vi "RotationApplication v5.vi"() -> ()   [LabVIEW 2012]
uses:
  <instrlib>/ZaberTSeries/Public/Utility/Request.ctl
  <instrlib>/ZaberTSeries/Public/Utility/Response.ctl
  <vilib>/Utility/file.llb/Write To Spreadsheet File (string).vi
  variables/GlobalUI.vi
  Stage Global.vi
  <instrlib>/ZaberTSeries/ZaberTSeries.lvlib
panel:
  out "Scanning?":bool
  out "Current Angle (deg)":dbl=45.0
  out "Stage Position (mm)":dbl=76.5
  in  "Time Step (ms)":dbl
  in  "Rotation f(x) (mm -> deg)":string="9.00000*x - 643.50000"
  in  "Finish Rotation f(x)":bool
  in  "Scan":bool
  in  "stop":bool
  in  "Go Home":bool
  in  "Set Home Offset":dbl=80.0
  in  "?":T1(tab)
  in  "Optimize":bool
  in  "Angle?":bool
  out "Current Angle (deg)":dbl=52.314375
  in  "Move Rel?":bool
  in  "Move Abs?":bool
  in  "Move Rel (deg)":dbl=-1.0 step=0.1
  in  "Move Abs (deg)":dbl=35.0
  in  "Send":bool
  out "Command?":bool=TRUE
  in  "REQUEST:":T2={"Device Number"=1, "Command"=23, "Data"=-10000, "Response Count"=1} {"Command" items=["Echo"=55, "Home"=1, "Move Absolute"=20, "Move Relative"=21, "Move at Constant Speed"=22, "Renumber"=2, "Restore Settings"=36, "Stop"=23]}
  out "Response Data:":T3 {"Command" items=["Constant Speed Tracking"=8, "Echo"=55, "Error"=255, "Home"=1, "Limit Active"=9, "Manual Move Tracking"=10, "Move Absolute"=20, "Move at Constant Speed"=22, "Move Relative"=21, "Renumber"=2, "Restore Settings"=36, "Stop"=23]}
  in  "Command":bool
  in  "DONE":bool
  in  "angle":dbl=7.89375
  in  "Aquire Data":bool
  out "Intensity vs Angle Plot":cluster{dbl[], dbl[]}(graph)={[0.1003125, 0.200625, 0.30093749999999997, 0.40125, 0.5015625, 0.6018749999999999, 0.7021875, 0.8025, 0.9028125, 1.003125, 1.1034374999999998, 1.2037499999999999, 1.3040625, 1.404375, 1.5046875, 1.605, 1.7053125, 1.805625, 1.9059374999999998, 2.00625, 2.1065625, 2.2068749999999997, 2.3071875, 2.4074999999999998, 2.5078125, 2.608125, 2.7084375, 2.80875, 2.9090625, 3.009375, 3.1096874999999997, 3.21, 3.3103124999999998, 3.410625, 3.5109375, 3.61125, 3.7115625, 3.8118749999999997, 3.9121875, 4.0125, 4.1128124999999995, 4.213125, 4.3134375, 4.413749999999999], [0.10330483041158461, 0.10354301638719464, 0.10354301638719464, 0.10358827172256029, 0.10358827172256029, 0.10288562309451152, 0.10288562309451152, 0.10288562309451152, 0.1017709127286577, 0.1017709127286577, 0.10044183498475528, 0.09877691501524301, 0.09877691501524301, 0.10001548208841382, 0.10001548208841382, 0.09941763528963352, 0.09941763528963352, 0.09897222751524294, 0.09965820312499914, 0.09965820312499914, 0.09993807164634047, 0.09985708841463325, 0.09985708841463325, 0.09985708841463325, 0.10042158917682856, 0.10075624047256009, 0.10075624047256009, 0.10102419969512122, 0.1007193216463409, 0.1007193216463409, 0.1007193216463409, 0.10111828315548696, 0.10111828315548696, 0.10111828315548696, 0.10066811166158449, 0.10066811166158449, 0.10040610708841394, 0.10110399199695043, 0.10110399199695043, 0.10115996570121859, 0.10115996570121859, 0.10151248094512112, 0.10151248094512112, 0.10125047637195043]}
  in  "Step Size (deg)":dbl=1.0
  in  "Final Angle (deg)":dbl=45.0
  in  "Initial Angle (deg)":dbl
  in  "Scan Angles":bool
  out "Calibrate?":bool
  in  "ABORT":bool
  in  "Simulation":bool
  out "Simulate?":bool
  in  "Finish Stage":bool
  in  "Start/pause":bool
  in  "Start/Pause Stage":bool
  out "Current Position (mm)":dbl
  in  "Finish Rotation":bool
  out "Current Angle":dbl
  in  "Initial Position (mm)":dbl
  in  "Final Position (mm)":dbl
  in  "Number of Steps":u32
  in  "Speed (um/s)":dbl
  in  "Final Angle (deg)":dbl=45.0
  in  "Number of Rotations":u32=4500
  in  "Polynomial Degree":dbl=1.0
  in  "VISA reference name:":refnum<visa-resource-name>="COM4"
  # "==>"
  # "Device"
  # "Command (Binary)"
  # "Data"
  # "==>"
  # "Data"
  # "==>"
  # "Rotation Mount Settings:"
  # "Simulated Delay Stage Settings:"
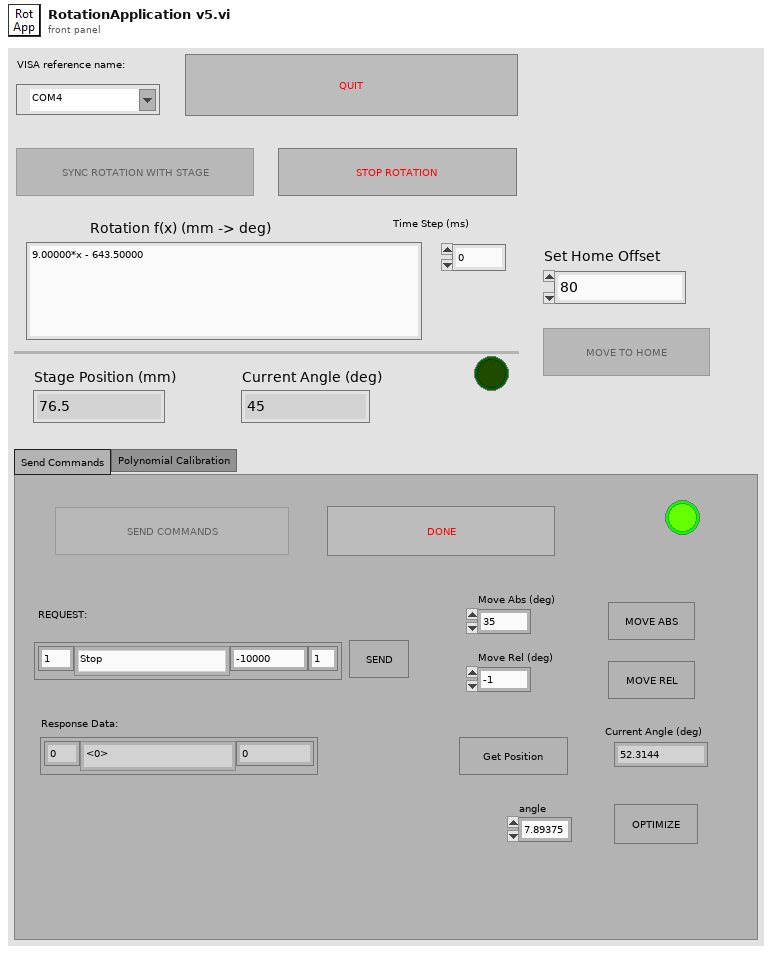
[diagram p1: front panel]
types:
  T1 = enum32{"Send Commands", "Polynomial Calibration", "Simulated f(x)  ", "Adjust Simulation Settings"}
  T2 = typedef "ZaberTSeries.lvlib/Request.ctl" = cluster{"Device Number":u8, "Command":u8, "Data":i32, "Response Count":i32}
  T3 = typedef "ZaberTSeries.lvlib/Response.ctl" = cluster{"Device Number":u8, "Command":u8, "Data":i32}
  T4 = enum8{"Enabled", "Disabled", "Disabled and Grayed Out"}
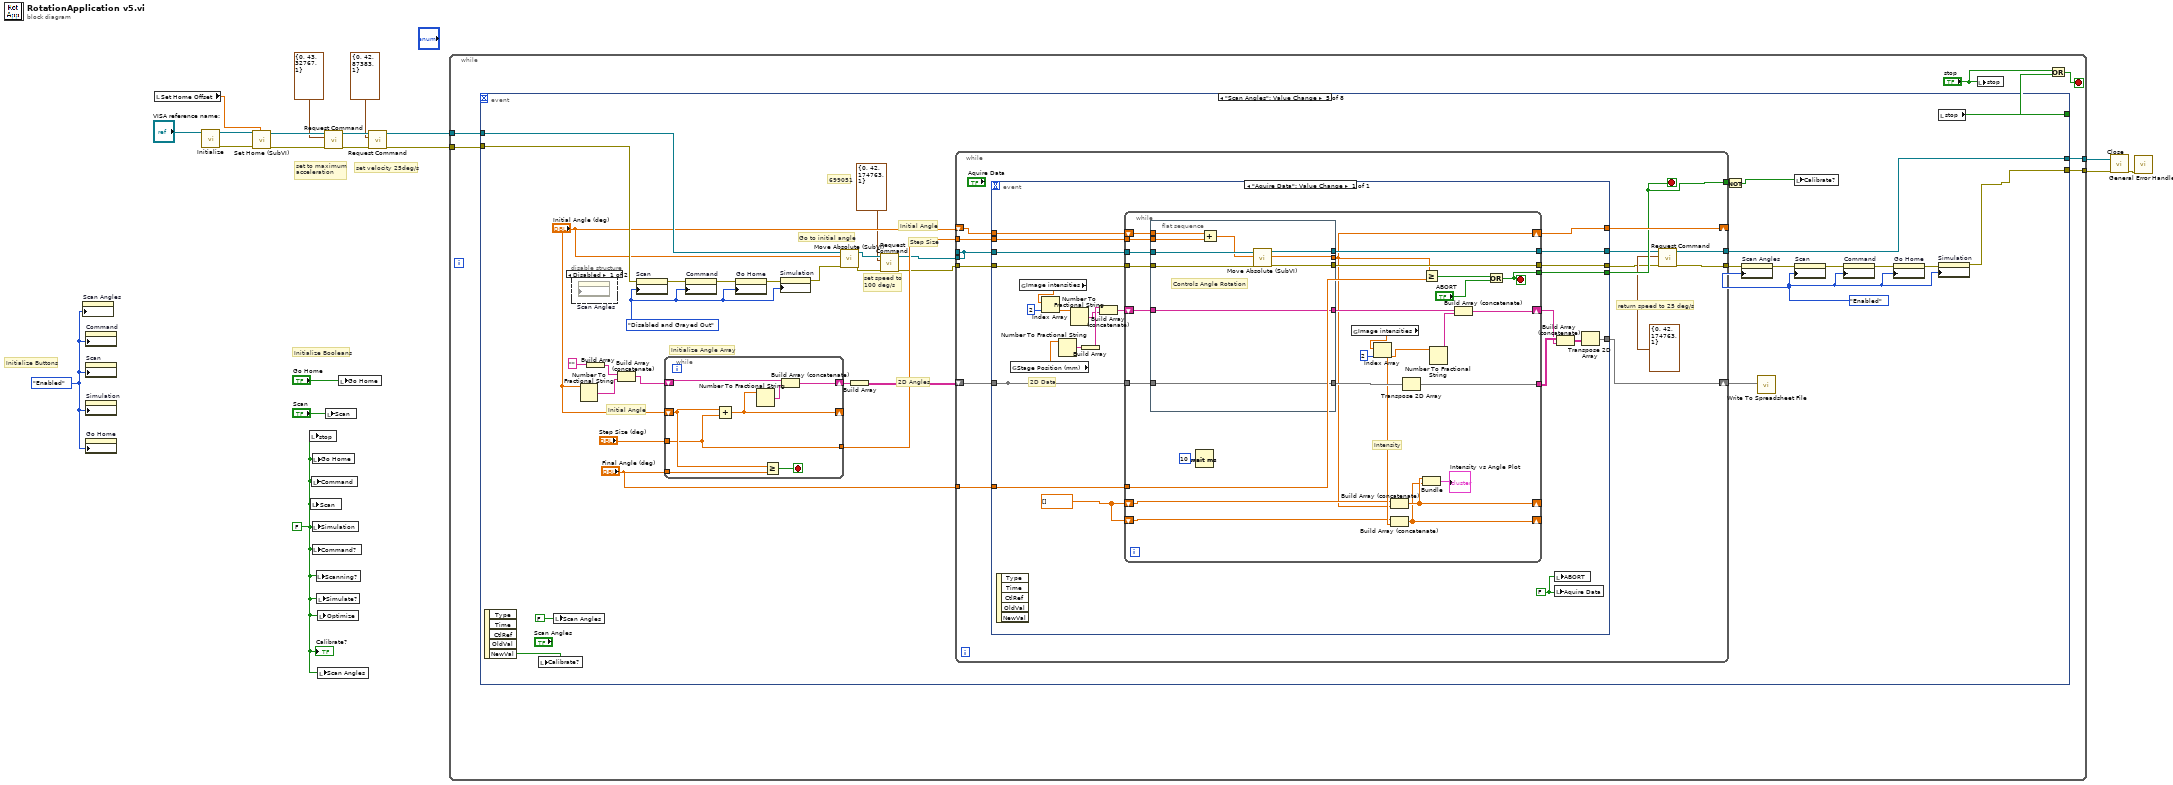
[diagram p0: block diagram]
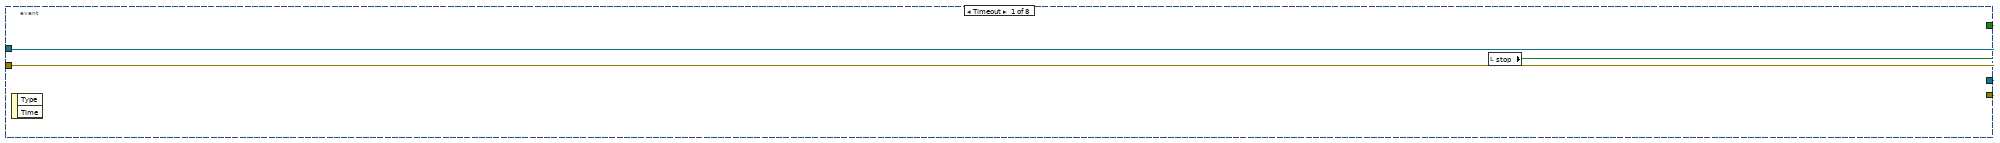
[diagram p2: hidden frame]
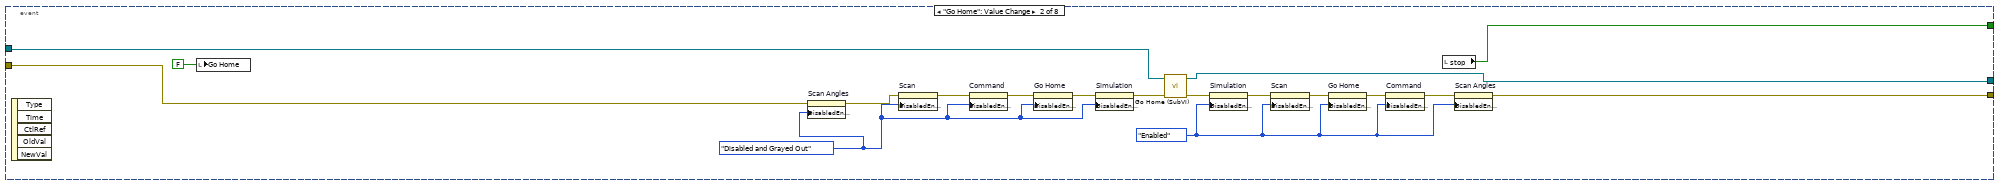
[diagram p3: hidden frame]
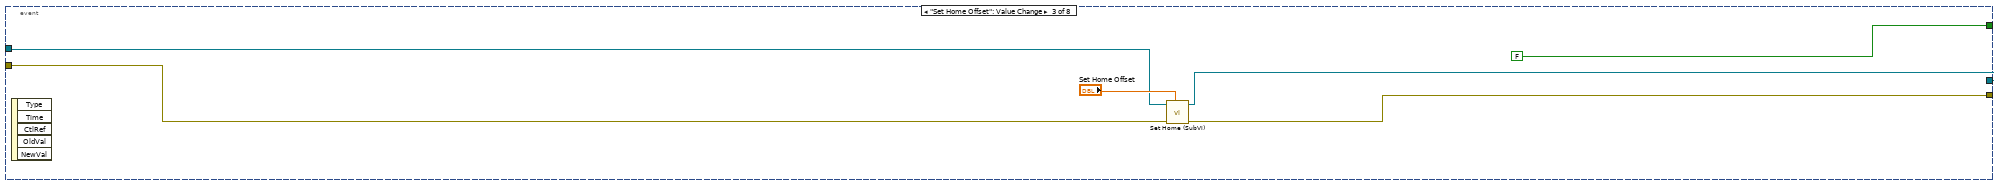
[diagram p4: hidden frame]
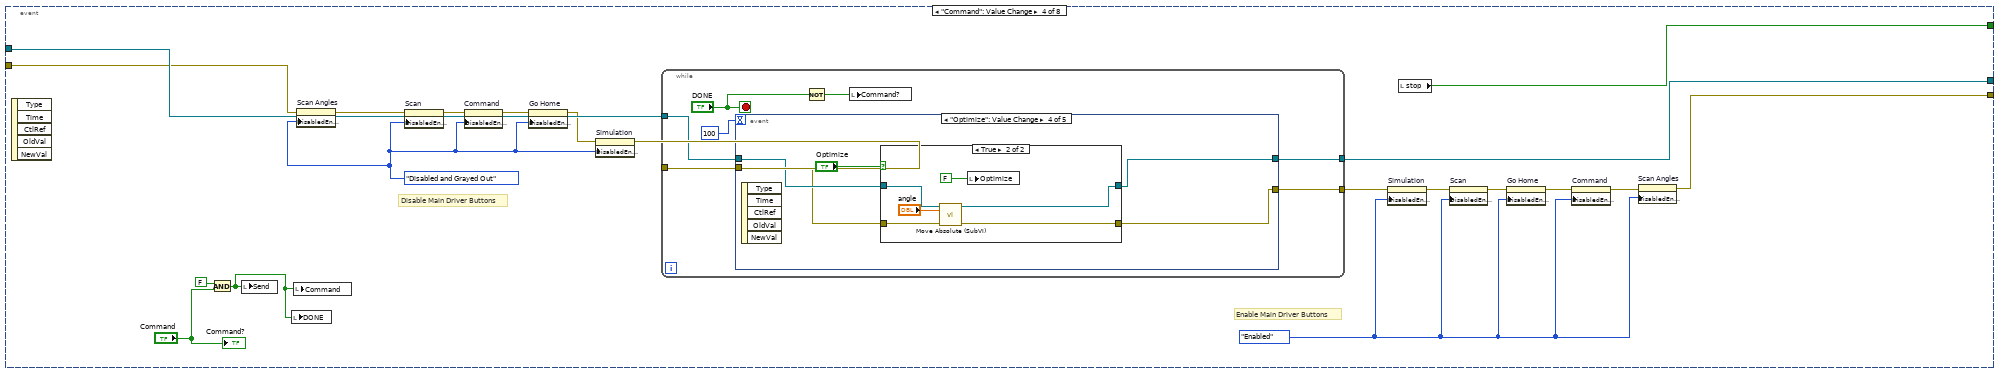
[diagram p5: hidden frame]
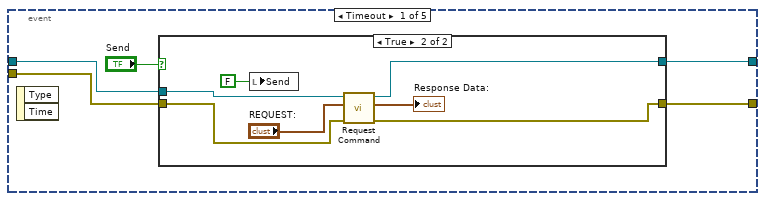
[diagram p6: hidden frame]
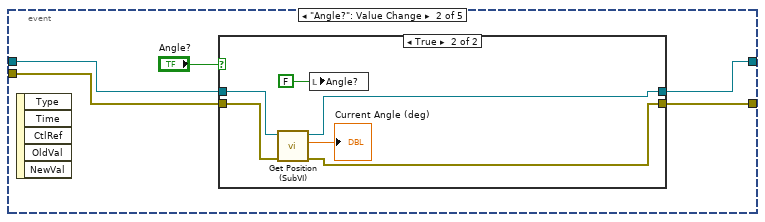
[diagram p8: hidden frame]
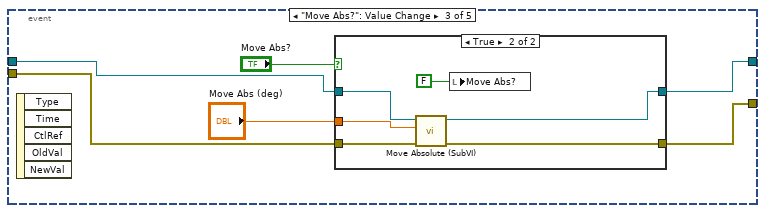
[diagram p10: hidden frame]
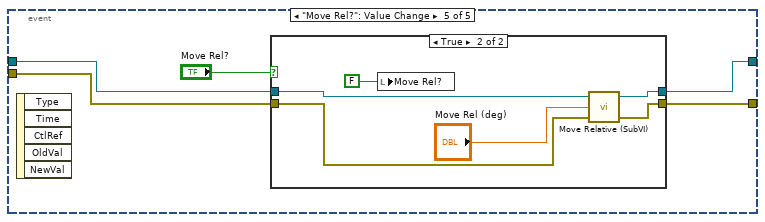
[diagram p13: hidden frame]
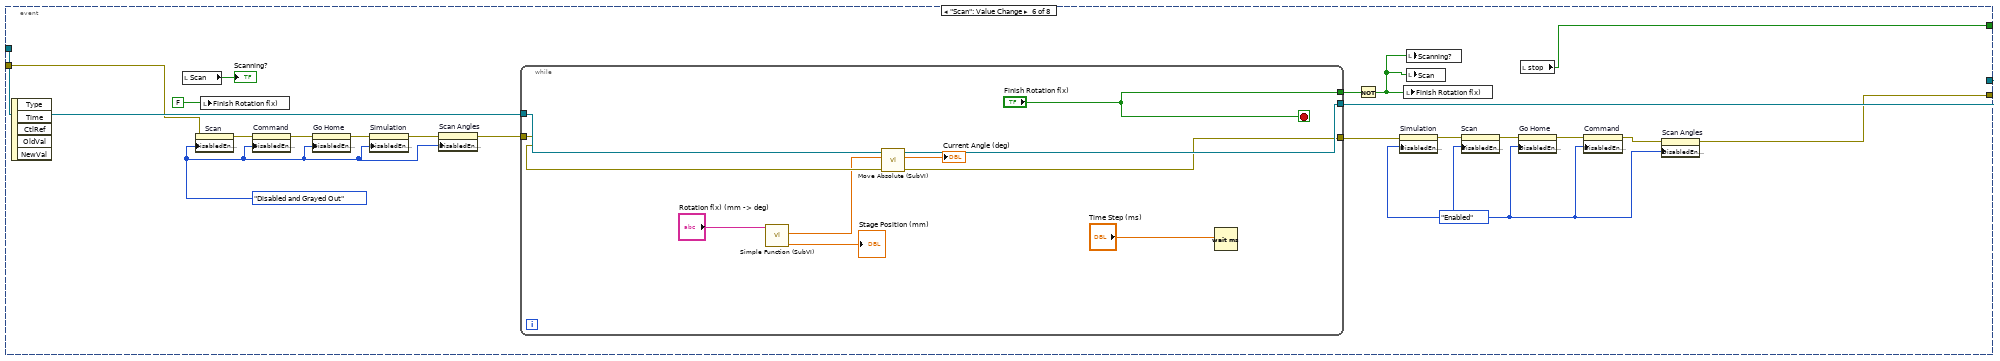
[diagram p16: hidden frame]
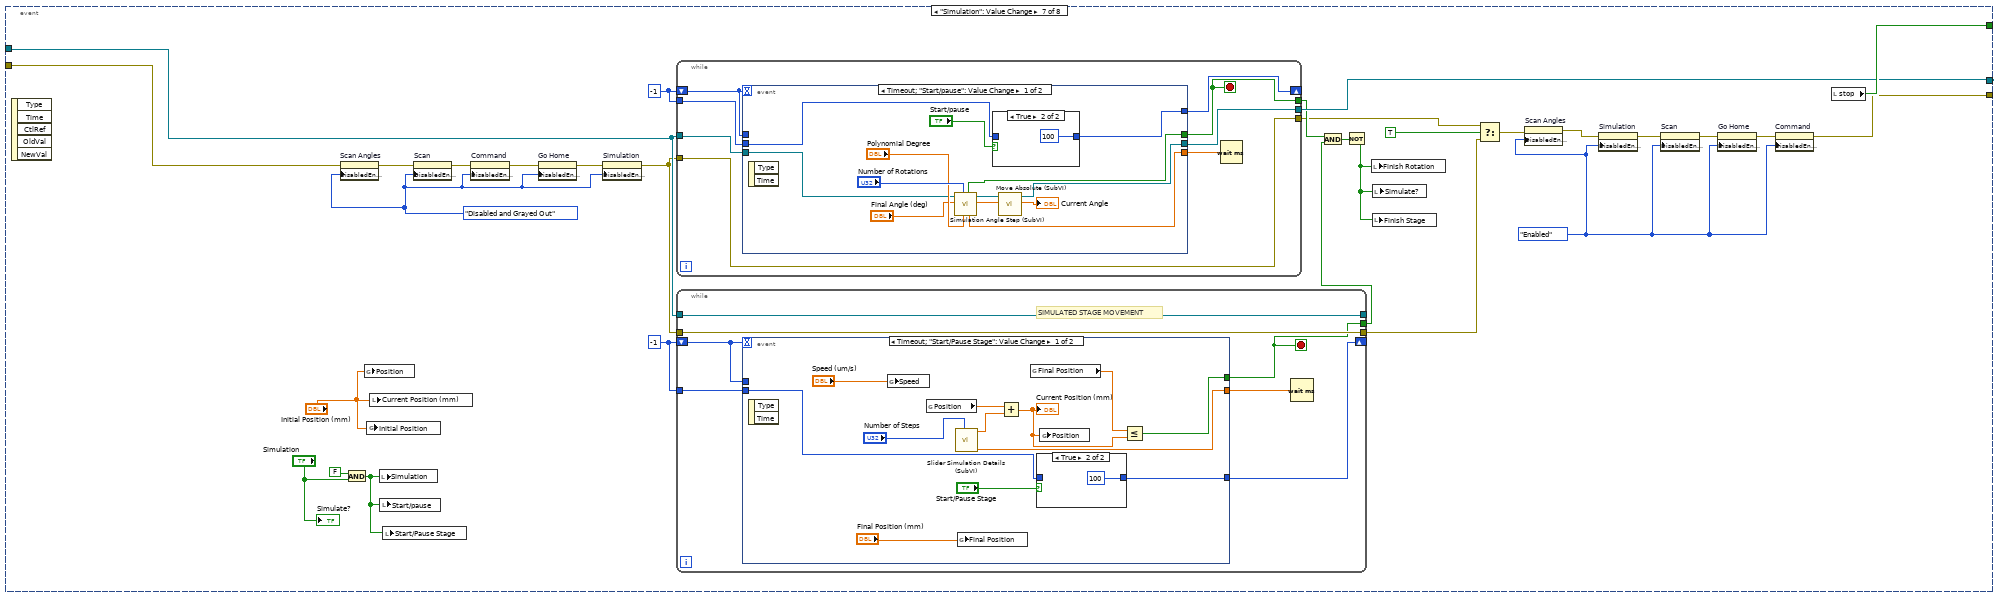
[diagram p17: hidden frame]
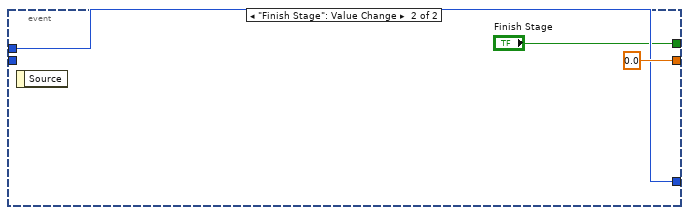
[diagram p19: hidden frame]
diagram:
  w9 = T4."Enabled" ("Disabled")
  w10 = FALSE ("y")
  # "set to maximum\nacceleration"
  # "set velocity 25deg/s"
  # "Initialize Buttons"
  # "Initialize Booleans"
  n1 = property on="Scan Angles" class="Bool (strict)"("DisabledEnum"=w9) -> ()  [unwired: 2 in, 2 out]
  n2 = property on="Command" class="Bool (strict)"("DisabledEnum"=w9) -> ()  [unwired: 2 in, 2 out]
  n3 = property on="Scan" class="Bool (strict)"("DisabledEnum"=w9) -> ()  [unwired: 2 in, 2 out]
  n4 = property on="Simulation" class="Bool (strict)"("DisabledEnum"=w9) -> ()  [unwired: 2 in, 2 out]
  n5 = property on="Go Home" class="Bool (strict)"("DisabledEnum"=w9) -> ()  [unwired: 2 in, 2 out]
  n6 = local read "Set Home Offset"() -> (w11:dbl)
  n7 = call <instrlib>:"Initialize.vi"("VISA resource name"="VISA reference name:") -> ("error out"=w12:errorcluster, "VISA resource name out"=w13:refnum<visa-resource-name>)  [unwired: 8 in, 1 out]
  n8 = call "Set Home (SubVI).vi"("Home Offset (deg)"=w11, "error in (no error)"=w12, "VISA Refnum in"=w13) -> ("error out"=w7:errorcluster, "VISA Refnum out"=w8:refnum<visa-resource-name>)  [unwired: 7 in]
  n9 = local write "stop"(w10) -> ()
  n10 = local write "Scan"(w10) -> ()
  n11 = local write "Command"(w10) -> ()
  n12 = local write "Go Home"(w10) -> ()
  n13 = local write "Simulation"(w10) -> ()
  n14 = local write "Command?"(w10) -> ()
  n15 = local write "Scanning?"(w10) -> ()
  n16 = local write "Simulate?"(w10) -> ()
  n17 = local write "Optimize"(w10) -> ()
  n18 = local write "Scan Angles"(w10) -> ()
  n19 = call <instrlib>:"Request Command.vi"("error in (no error)"=w7, "Request"=T2 {"Device Number"=0, "Command"=43, "Data"=32767, "Response Count"=1}, "VISA resource name"=w8) -> ("error out"=w5:errorcluster, "VISA resource name out"=w6:refnum<visa-resource-name>)  [unwired: 5 in, 2 out]
  n20 = local write "Scan"("Scan") -> ()
  n21 = local write "Go Home"("Go Home") -> ()
  n22 = call <instrlib>:"Request Command.vi"("error in (no error)"=w5, "Request"=T2 {"Device Number"=0, "Command"=42, "Data"=87383, "Response Count"=1}, "VISA resource name"=w6) -> ("error out"=w3:errorcluster, "VISA resource name out"=w4:refnum<visa-resource-name>)  [unwired: 5 in, 2 out]
  n23 = while {
    tunnel: w4 -> [w23]
    tunnel: w3 -> [w22]
    tunnel: [w26] -> w17
    tunnel: [w25] -> w19
    stop <- w24 stop-if-true
    n24 = event shown="[4] \"Scan Angles\": Value Change" {
      selector: _ -> [_ _ _ _ _ _ _ _]
      dyn-events: _ -> [_ _ _ _ _ _ _ _]
      timeout: _ -> [_ _ _ _ _ _ _ _]
      tunnel: w23 -> [w29 w42 w52 w73 w173 w286 w316 w380]
      tunnel: w22 -> [w28 w33 w51 w59 w177 w283 w301 w379]
      tunnel: [w29 w37 w50 w65 w148 w285 w323 w380] -> w25
      tunnel: [w28 w30 w49 w54 w149 w267 w320 w379] -> w26
      tunnel: [w27 w47 FALSE ("stop") w72 w183 w287 w327 w381] -> w21
      event Timeout {
        n25 = event-data() -> ()  [unwired: 1 in, 2 out]
        n26 = local read "stop"() -> (w27:bool)
      }
      event "Go Home": Value Change {
        w31 = T4."Enabled" ("Disabled")
        w35 = T4."Disabled and Grayed Out" ("Disabled")
        n27 = event-data() -> ()  [unwired: 1 in, 5 out]
        n28 = local write "Go Home"(FALSE ("Go Home")) -> ()
        n29 = property on="Scan Angles" class="Bool (strict)"(error in=w33, "DisabledEnum"=w35) -> (error out=w34:errorcluster)  [unwired: 1 in, 1 out]
        n30 = property on="Scan" class="Bool (strict)"(error in=w34, "DisabledEnum"=w35) -> (error out=w45:errorcluster)  [unwired: 1 in, 1 out]
        n31 = property on="Command" class="Bool (strict)"(error in=w45, "DisabledEnum"=w35) -> (error out=w44:errorcluster)  [unwired: 1 in, 1 out]
        n32 = property on="Go Home" class="Bool (strict)"(error in=w44, "DisabledEnum"=w35) -> (error out=w43:errorcluster)  [unwired: 1 in, 1 out]
        n33 = property on="Simulation" class="Bool (strict)"(error in=w43, "DisabledEnum"=w35) -> (error out=w41:errorcluster)  [unwired: 1 in, 1 out]
        n34 = call "Go Home (SubVI).vi"("error in (no error)"=w41, "VISA Refnum in"=w42) -> ("error out"=w36:errorcluster, "VISA Refnum out"=w37:refnum<visa-resource-name>)  [unwired: 8 in]
        n35 = property on="Simulation" class="Bool (strict)"(error in=w36, "DisabledEnum"=w31) -> (error out=w38:errorcluster)  [unwired: 1 in, 1 out]
        n36 = property on="Scan" class="Bool (strict)"(error in=w38, "DisabledEnum"=w31) -> (error out=w40:errorcluster)  [unwired: 1 in, 1 out]
        n37 = property on="Go Home" class="Bool (strict)"(error in=w40, "DisabledEnum"=w31) -> (error out=w39:errorcluster)  [unwired: 1 in, 1 out]
        n38 = property on="Command" class="Bool (strict)"(error in=w39, "DisabledEnum"=w31) -> (error out=w32:errorcluster)  [unwired: 1 in, 1 out]
        n39 = local read "stop"() -> (w47:bool)
        n40 = property on="Scan Angles" class="Bool (strict)"(error in=w32, "DisabledEnum"=w31) -> (error out=w30:errorcluster)  [unwired: 1 in, 1 out]
      }
      event "Set Home Offset": Value Change {
        n41 = event-data() -> ()  [unwired: 1 in, 5 out]
        n42 = call "Set Home (SubVI).vi"("Home Offset (deg)"="Set Home Offset", "error in (no error)"=w51, "VISA Refnum in"=w52) -> ("error out"=w49:errorcluster, "VISA Refnum out"=w50:refnum<visa-resource-name>)  [unwired: 7 in]
      }
      event "Command": Value Change {
        w56 = T4."Enabled" ("Disabled")
        w57 = T4."Disabled and Grayed Out" ("Disabled")
        # "Enable Main Driver Buttons"
        # "Disable Main Driver Buttons"
        n43 = event-data() -> ()  [unwired: 1 in, 5 out]
        n44 = And(x=FALSE ("Command"), y="Command") -> (x .and. y?=w61:bool)
        n45 = local write "Send"(w61) -> ()
        n46 = local write "DONE"(w61) -> ()
        n47 = local write "Command"(w61) -> ()
        n48 = property on="Scan Angles" class="Bool (strict)"(error in=w59, "DisabledEnum"=w57) -> (error out=w58:errorcluster)  [unwired: 1 in, 1 out]
        n49 = property on="Scan" class="Bool (strict)"(error in=w58, "DisabledEnum"=w57) -> (error out=w67:errorcluster)  [unwired: 1 in, 1 out]
        n50 = property on="Command" class="Bool (strict)"(error in=w67, "DisabledEnum"=w57) -> (error out=w68:errorcluster)  [unwired: 1 in, 1 out]
        n51 = property on="Go Home" class="Bool (strict)"(error in=w68, "DisabledEnum"=w57) -> (error out=w69:errorcluster)  [unwired: 1 in, 1 out]
        n52 = property on="Simulation" class="Bool (strict)"(error in=w69, "DisabledEnum"=w57) -> (error out=w66:errorcluster)  [unwired: 1 in, 1 out]
        n53 = while {
          tunnel: w73 -> [w76]
          tunnel: [w80] -> w65
          tunnel: w66 -> [w75]
          tunnel: [w79] -> w60
          stop <- "DONE" stop-if-true
          n54 = event shown="[3] \"Optimize\": Value Change" {
            selector: _ -> [_ _ _ _ _]
            dyn-events: _ -> [_ _ _ _ _]
            timeout: 100 -> [_ _ _ _ _]
            tunnel: [w85 w98 w110 w123 w136] -> w80
            tunnel: [w84 w95 w108 w122 w135] -> w79
            tunnel: w76 -> [w82 w97 w111 w125 w138]
            tunnel: w75 -> [w81 w96 w109 w124 w137]
            event Timeout {
              n55 = event-data() -> ()  [unwired: 1 in, 2 out]
              n56 = case shown="True" "Send" {
                tunnel: w82 -> [w87 w93]
                tunnel: [w87 w92] -> w85
                tunnel: w81 -> [w86 w91]
                tunnel: [w86 w90] -> w84
                frame False {
                }
                frame True {
                  n57 = local write "Send"(FALSE ("Send")) -> ()
                  n58 = call <instrlib>:"Request Command.vi"("error in (no error)"=w91, "Request"="REQUEST:", "VISA resource name"=w93) -> ("error out"=w90:errorcluster, "First Response"=→"Response Data:":T3, "VISA resource name out"=w92:refnum<visa-resource-name>)  [unwired: 5 in, 1 out]
                }
              }
            }
            event "Angle?": Value Change {
              n59 = event-data() -> ()  [unwired: 1 in, 5 out]
              n60 = case shown="True" "Angle?" {
                tunnel: [w101 w106] -> w98
                tunnel: w97 -> [w101 w105]
                tunnel: w96 -> [w100 w104]
                tunnel: [w100 w103] -> w95
                frame False {
                }
                frame True {
                  n61 = call "Get Position (SubVI).vi"("error in (no error)"=w104, "VISA Refnum in"=w105) -> ("error out"=w103:errorcluster, "Position"=→"Current Angle (deg)":dbl, "VISA Refnum out"=w106:refnum<visa-resource-name>)  [unwired: 7 in]
                  n62 = local write "Angle?"(FALSE ("Angle?")) -> ()
                }
              }
            }
            event "Move Abs?": Value Change {
              n63 = event-data() -> ()  [unwired: 1 in, 5 out]
              n64 = case shown="True" "Move Abs?" {
                tunnel: "Move Abs (deg)" -> [_ w117]
                tunnel: w111 -> [w115 w121]
                tunnel: [w115 w120] -> w110
                tunnel: w109 -> [w114 w119]
                tunnel: [w114 w118] -> w108
                frame False {
                }
                frame True {
                  n65 = call "Move Absolute (SubVI).vi"("error in (no error)"=w119, "Move to Angle"=w117, "VISA Refnum in"=w121) -> ("error out"=w118:errorcluster, "VISA Refnum out"=w120:refnum<visa-resource-name>)  [unwired: 6 in, 1 out]
                  n66 = local write "Move Abs?"(FALSE ("Move Abs?")) -> ()
                }
              }
            }
            event "Optimize": Value Change {
              n67 = event-data() -> ()  [unwired: 1 in, 5 out]
              n68 = case shown="True" "Optimize" {
                tunnel: w125 -> [w128 w134]
                tunnel: [w128 w133] -> w123
                tunnel: w124 -> [w127 w132]
                tunnel: [w127 w131] -> w122
                frame False {
                }
                frame True {
                  n69 = call "Move Absolute (SubVI).vi"("error in (no error)"=w132, "Move to Angle"="angle", "VISA Refnum in"=w134) -> ("error out"=w131:errorcluster, "VISA Refnum out"=w133:refnum<visa-resource-name>)  [unwired: 6 in, 1 out]
                  n70 = local write "Optimize"(FALSE ("Move Abs?")) -> ()
                }
              }
            }
            event "Move Rel?": Value Change {
              n71 = event-data() -> ()  [unwired: 1 in, 5 out]
              n72 = case shown="True" "Move Rel?" {
                tunnel: w138 -> [w141 w146]
                tunnel: w137 -> [w140 w145]
                tunnel: [w141 w143] -> w136
                tunnel: [w140 w144] -> w135
                frame False {
                }
                frame True {
                  n73 = local write "Move Rel?"(FALSE ("Move Rel?")) -> ()
                  n74 = call "Move Relative (SubVI).vi"("error in (no error)"=w145, "Degrees to move"="Move Rel (deg)", "VISA resource name"=w146) -> ("error out"=w144:errorcluster, "VISA resource name out"=w143:refnum<visa-resource-name>)  [unwired: 1 out]
                }
              }
            }
          }
          n75 = Not(x="DONE") -> (.not. x?=w77:bool)
          n76 = local write "Command?"(w77) -> ()
        }
        n77 = property on="Simulation" class="Bool (strict)"(error in=w60, "DisabledEnum"=w56) -> (error out=w62:errorcluster)  [unwired: 1 in, 1 out]
        n78 = local read "stop"() -> (w72:bool)
        n79 = property on="Scan" class="Bool (strict)"(error in=w62, "DisabledEnum"=w56) -> (error out=w64:errorcluster)  [unwired: 1 in, 1 out]
        n80 = property on="Go Home" class="Bool (strict)"(error in=w64, "DisabledEnum"=w56) -> (error out=w63:errorcluster)  [unwired: 1 in, 1 out]
        n81 = property on="Command" class="Bool (strict)"(error in=w63, "DisabledEnum"=w56) -> (error out=w55:errorcluster)  [unwired: 1 in, 1 out]
        n82 = property on="Scan Angles" class="Bool (strict)"(error in=w55, "DisabledEnum"=w56) -> (error out=w54:errorcluster)  [unwired: 1 in, 1 out]
        "Command?" <- "Command"
      }
      event "Scan Angles": Value Change {
        w169 = T4."Enabled" ("Disabled")
        w170 = T4."Disabled and Grayed Out" ("Disabled")
        # "699051"
        # "set speed to\n100 deg/s"
        # "Initial Angle"
        # "2D Angles"
        # "Go to initial angle"
        # "Step Size"
        # "Initial Angle"
        # "Initialize Angle Array"
        n83 = event-data() -> ("NewVal"=w182:bool)  [unwired: 1 in, 4 out]
        n84 = local write "Calibrate?"(w182) -> ()
        n85 = local write "Scan Angles"(FALSE ("Scan Angles")) -> ()
        n86 = disable-structure shown="Disabled" {
          frame Disabled {
            n87 = property on="Scan Angles" class="Bool (strict)" props=["DisabledEnum"]() -> ()  [unwired: 3 in, 2 out]
          }
          frame Enabled {
          }
        }
        n88 = Number To Fractional String(number="Initial Angle (deg)") -> (F-format string=w163:string)  [unwired: 3 in]
        n89 = Build Array("") -> (w164:string[])
        n90 = Build Array (concatenate)(w164, w163) -> (w162:string[])
        n91 = property on="Scan" class="Bool (strict)"(error in=w177, "DisabledEnum"=w170) -> (error out=w179:errorcluster)  [unwired: 1 in, 1 out]
        n92 = while {
          tunnel: [w184] -> w167
          shift-right: [w185] -> _
          shift-left: "Initial Angle (deg)" -> [w189]
          tunnel: "Final Angle (deg)" -> [w190]
          shift-right: [w187] -> w161
          shift-left: w162 -> [w188]
          tunnel: "Step Size (deg)" -> [w184]
          stop <- w191 stop-if-true
          n93 = Add(x=w189, y=w184) -> (x+y=w185:dbl)
          n94 = Number To Fractional String(number=w185) -> (F-format string=w186:string)  [unwired: 3 in]
          n95 = Greater Or Equal?(x=w189, y=w190) -> (x >= y?=w191:bool)
          n96 = Build Array (concatenate)(w188, w186) -> (w187:string[])
        }
        n97 = property on="Command" class="Bool (strict)"(error in=w179, "DisabledEnum"=w170) -> (error out=w180:errorcluster)  [unwired: 1 in, 1 out]
        n98 = property on="Go Home" class="Bool (strict)"(error in=w180, "DisabledEnum"=w170) -> (error out=w178:errorcluster)  [unwired: 1 in, 1 out]
        n99 = property on="Simulation" class="Bool (strict)"(error in=w178, "DisabledEnum"=w170) -> (error out=w172:errorcluster)  [unwired: 1 in, 1 out]
        n100 = call "Move Absolute (SubVI).vi"("error in (no error)"=w172, "Move to Angle"="Initial Angle (deg)", "VISA Refnum in"=w173) -> ("error out"=w151:errorcluster, "VISA Refnum out"=w154:refnum<visa-resource-name>)  [unwired: 6 in, 1 out]
        n101 = Build Array(w161) -> (w160:string[][])
        n102 = call <instrlib>:"Request Command.vi"("error in (no error)"=w151, "Request"=T2 {"Device Number"=0, "Command"=42, "Data"=174763, "Response Count"=1}, "VISA resource name"=w154) -> ("error out"=w152:errorcluster, "VISA resource name out"=w153:refnum<visa-resource-name>)  [unwired: 5 in, 2 out]
        n103 = while {
          tunnel: w167 -> [w205]
          tunnel: "Final Angle (deg)" -> [w203]
          tunnel: w152 -> [w204]
          tunnel: [w197] -> _
          tunnel: [w193] -> w168
          tunnel: [w194] -> w148
          shift-right: [w201] -> _
          shift-left: "Initial Angle (deg)" -> [w202]
          shift-right: [w199] -> w159
          shift-left: w160 -> [w200]
          tunnel: [w198] -> w157
          tunnel: w153 -> [w197]
          stop <- w198 stop-if-true
          # "return speed to 25 deg/s"
          n104 = event shown="[0] \"Aquire Data\": Value Change" {
            selector: _ -> [_]
            dyn-events: _ -> [_]
            timeout: _ -> [_]
            tunnel: w205 -> [w229]
            tunnel: w197 -> [w228]
            tunnel: w204 -> [w227]
            tunnel: [w226] -> w195
            tunnel: [w225] -> w192
            tunnel: w203 -> [w224]
            tunnel: w202 -> [w207]
            tunnel: [w223] -> w201
            tunnel: [w222] -> _
            tunnel: w200 -> [w222]
            tunnel: [w215] -> w199
            tunnel: [w206] -> w198
            event "Aquire Data": Value Change {
              w208 = dbl[] []
              w214 = FALSE ("Aquire Data")
              # "2D Data"
              n105 = event-data() -> ()  [unwired: 1 in, 5 out]
              n106 = global read "GlobalUI.vi" "Stage Position (mm)"() -> (w213:dbl)
              n107 = global read "GlobalUI.vi" "Image intensities"() -> (w221:dbl[])
              n108 = Index Array(array=w221, index=2) -> (element=w218:dbl)
              n109 = Number To Fractional String(number=w213) -> (F-format string=w212:string)  [unwired: 3 in]
              n110 = Number To Fractional String(number=w218) -> (F-format string=w210:string)  [unwired: 3 in]
              n111 = Build Array(w212) -> (w211:string[])
              n112 = Build Array (concatenate)(w211, w210) -> (w209:string[])
              n113 = while {
                tunnel: w229 -> [w256]
                tunnel: w228 -> [w255]
                tunnel: w227 -> [w254]
                tunnel: [w253] -> w226
                tunnel: [w252] -> w225
                tunnel: w224 -> [w251]
                tunnel: w222 -> [w241]
                shift-right: [w246] -> w217
                shift-left: w209 -> [w243]
                tunnel: [w245] -> w219
                shift-right: [w235] -> _
                shift-left: w208 -> [w238]
                shift-right: [w236] -> _
                shift-left: w208 -> [w237]
                shift-right: [w233] -> w223
                shift-left: w207 -> [w232]
                tunnel: [w231] -> w206
                stop <- w231 stop-if-true
                # "Intensity"
                n114 = flat-sequence {
                  tunnel: w256 -> [w257]
                  tunnel: w255 -> [w266]
                  tunnel: w254 -> [w265]
                  tunnel: [w264] -> w253
                  tunnel: [w263] -> w252
                  tunnel: w232 -> [w258]
                  tunnel: w243 -> [w261]
                  tunnel: [w261] -> w242
                  tunnel: w241 -> [w260]
                  tunnel: [w260] -> w240
                  tunnel: [w259] -> w233
                  frame #0 {
                    # "Controls Angle Rotation"
                    n115 = Add(x=w258, y=w257) -> (x+y=w262:dbl)
                    n116 = call "Move Absolute (SubVI).vi"("error in (no error)"=w265, "Move to Angle"=w262, "VISA Refnum in"=w266) -> ("error out"=w263:errorcluster, "New Angle"=w259:dbl, "VISA Refnum out"=w264:refnum<visa-resource-name>)  [unwired: 6 in]
                  }
                }
                n117 = Wait (ms)(milliseconds to wait=u32 10) -> ()  [unwired: 1 out]
                n118 = global read "GlobalUI.vi" "Image intensities"() -> (w248:dbl[])
                n119 = Index Array(array=w248, index=2) -> (element=w239:dbl)
                n120 = Build Array (concatenate)(w238, w239) -> (w235:dbl[])
                n121 = Build Array (concatenate)(w237, w233) -> (w236:dbl[])
                n122 = Transpose 2D Array(2D array=w240) -> (transposed array=w245:string[][])
                n123 = Greater Or Equal?(x=w233, y=w251) -> (x >= y?=w249:bool)
                n124 = Bundle(w236, w235) -> (→"Intensity vs Angle Plot":cluster{dbl[], dbl[]})  [unwired: 1 in]
                n125 = Number To Fractional String(number=w239) -> (F-format string=w244:string)  [unwired: 3 in]
                n126 = Build Array (concatenate)(w242, w244) -> (w246:string[])
                n127 = Or(x=w249, y="ABORT") -> (x .or. y?=w231:bool)
              }
              n128 = local write "Aquire Data"(w214) -> ()
              n129 = local write "ABORT"(w214) -> ()
              n130 = Build Array (concatenate)(w219, w217) -> (w216:string[][])
              n131 = Transpose 2D Array(2D array=w216) -> (transposed array=w215:string[][])
            }
          }
          n132 = call <instrlib>:"Request Command.vi"("error in (no error)"=w192, "Request"=T2 {"Device Number"=0, "Command"=42, "Data"=174763, "Response Count"=1}, "VISA resource name"=w195) -> ("error out"=w193:errorcluster, "VISA resource name out"=w194:refnum<visa-resource-name>)  [unwired: 5 in, 2 out]
        }
        n133 = Not(x=w157) -> (.not. x?=w156:bool)
        n134 = property on="Scan Angles" class="Bool (strict)"(error in=w168, "DisabledEnum"=w169) -> (error out=w155:errorcluster)  [unwired: 1 in, 1 out]
        n135 = call-poly <vilib>:"Write To Spreadsheet File.vi"("2D data"=w159) -> ()  [unwired: 7 in, 1 out]
        n136 = local write "Calibrate?"(w156) -> ()
        n137 = property on="Scan" class="Bool (strict)"(error in=w155, "DisabledEnum"=w169) -> (error out=w175:errorcluster)  [unwired: 1 in, 1 out]
        n138 = property on="Command" class="Bool (strict)"(error in=w175, "DisabledEnum"=w169) -> (error out=w176:errorcluster)  [unwired: 1 in, 1 out]
        n139 = property on="Go Home" class="Bool (strict)"(error in=w176, "DisabledEnum"=w169) -> (error out=w174:errorcluster)  [unwired: 1 in, 1 out]
        n140 = property on="Simulation" class="Bool (strict)"(error in=w174, "DisabledEnum"=w169) -> (error out=w149:errorcluster)  [unwired: 1 in, 1 out]
        n141 = local read "stop"() -> (w183:bool)
      }
      event "Scan": Value Change {
        w268 = T4."Enabled" ("Disabled")
        w270 = T4."Disabled and Grayed Out" ("Disabled")
        n142 = event-data() -> ()  [unwired: 1 in, 5 out]
        n143 = local read "Scan"() -> (→"Scanning?":bool)
        n144 = property on="Scan" class="Bool (strict)"(error in=w283, "DisabledEnum"=w270) -> (error out=w282:errorcluster)  [unwired: 1 in, 1 out]
        n145 = local write "Finish Rotation f(x)"(FALSE ("Command")) -> ()
        n146 = property on="Command" class="Bool (strict)"(error in=w282, "DisabledEnum"=w270) -> (error out=w284:errorcluster)  [unwired: 1 in, 1 out]
        n147 = property on="Go Home" class="Bool (strict)"(error in=w284, "DisabledEnum"=w270) -> (error out=w279:errorcluster)  [unwired: 1 in, 1 out]
        n148 = property on="Simulation" class="Bool (strict)"(error in=w279, "DisabledEnum"=w270) -> (error out=w272:errorcluster)  [unwired: 1 in, 1 out]
        n149 = property on="Scan Angles" class="Bool (strict)"(error in=w272, "DisabledEnum"=w270) -> (error out=w271:errorcluster)  [unwired: 1 in, 1 out]
        n150 = while {
          tunnel: w286 -> [w297]
          tunnel: [w296] -> w285
          tunnel: w271 -> [w295]
          tunnel: [w294] -> w277
          tunnel: ["Finish Rotation f(x)"] -> w273
          stop <- "Finish Rotation f(x)" stop-if-true
          n151 = call "Simple Function (SubVI).vi"("f(x) (mm -> deg)"="Rotation f(x) (mm -> deg)") -> ("Stage Position (mm)"=→"Stage Position (mm)":dbl, "Next Angle (deg)"=w291:dbl)  [unwired: 9 in]
          n152 = call "Move Absolute (SubVI).vi"("error in (no error)"=w295, "Move to Angle"=w291, "VISA Refnum in"=w297) -> ("error out"=w294:errorcluster, "New Angle"=→"Current Angle (deg)":dbl, "VISA Refnum out"=w296:refnum<visa-resource-name>)  [unwired: 6 in]
          n153 = Wait (ms)(milliseconds to wait="Time Step (ms)") -> ()  [unwired: 1 out]
        }
        n154 = Not(x=w273) -> (.not. x?=w274:bool)
        n155 = property on="Simulation" class="Bool (strict)"(error in=w277, "DisabledEnum"=w268) -> (error out=w278:errorcluster)  [unwired: 1 in, 1 out]
        n156 = local write "Finish Rotation f(x)"(w274) -> ()
        n157 = local write "Scanning?"(w274) -> ()
        n158 = local write "Scan"(w274) -> ()
        n159 = property on="Scan" class="Bool (strict)"(error in=w278, "DisabledEnum"=w268) -> (error out=w280:errorcluster)  [unwired: 1 in, 1 out]
        n160 = property on="Go Home" class="Bool (strict)"(error in=w280, "DisabledEnum"=w268) -> (error out=w281:errorcluster)  [unwired: 1 in, 1 out]
        n161 = local read "stop"() -> (w287:bool)
        n162 = property on="Command" class="Bool (strict)"(error in=w281, "DisabledEnum"=w268) -> (error out=w269:errorcluster)  [unwired: 1 in, 1 out]
        n163 = property on="Scan Angles" class="Bool (strict)"(error in=w269, "DisabledEnum"=w268) -> (error out=w267:errorcluster)  [unwired: 1 in, 1 out]
      }
      event "Simulation": Value Change {
        w310 = -1
        w309 = -1
        w300 = T4."Enabled" ("Disabled")
        w303 = T4."Disabled and Grayed Out" ("Disabled")
        n164 = event-data() -> ()  [unwired: 1 in, 5 out]
        n165 = property on="Scan Angles" class="Bool (strict)"(error in=w301, "DisabledEnum"=w303) -> (error out=w302:errorcluster)  [unwired: 1 in, 1 out]
        n166 = And(x=FALSE ("Command"), y="Simulation") -> (x .and. y?=w304:bool)
        n167 = global write "Stage Global.vi" "Position"("Initial Position (mm)") -> ()
        n168 = global write "Stage Global.vi" "Initial Position"("Initial Position (mm)") -> ()
        n169 = local write "Current Position (mm)"("Initial Position (mm)") -> ()
        n170 = local write "Simulation"(w304) -> ()
        n171 = local write "Start/pause"(w304) -> ()
        n172 = local write "Start/Pause Stage"(w304) -> ()
        n173 = property on="Scan" class="Bool (strict)"(error in=w302, "DisabledEnum"=w303) -> (error out=w326:errorcluster)  [unwired: 1 in, 1 out]
        n174 = property on="Command" class="Bool (strict)"(error in=w326, "DisabledEnum"=w303) -> (error out=w325:errorcluster)  [unwired: 1 in, 1 out]
        n175 = property on="Go Home" class="Bool (strict)"(error in=w325, "DisabledEnum"=w303) -> (error out=w324:errorcluster)  [unwired: 1 in, 1 out]
        n176 = property on="Simulation" class="Bool (strict)"(error in=w324, "DisabledEnum"=w303) -> (error out=w315:errorcluster)  [unwired: 1 in, 1 out]
        n177 = while {
          tunnel: w315 -> [w359]
          tunnel: w316 -> [w354]
          tunnel: [w353] -> w323
          tunnel: [w359] -> w306
          tunnel: [w358] -> w312
          shift-right: [w357] -> _
          shift-left: w310 -> [w355]
          tunnel: w310 -> [w356]
          stop <- w358 stop-if-true
          n178 = event shown="[0] Timeout;  \"Start/pause\": Value Change" {
            selector: _ -> [_ _]
            dyn-events: _ -> [_ _]
            timeout: w355 -> [_ _]
            tunnel: [w360 "Finish Rotation"] -> w358
            tunnel: [w371 w377] -> w357
            tunnel: w356 -> [w370 _]
            tunnel: w355 -> [_ w377]
            tunnel: w354 -> [w365 w376]
            tunnel: [w364 w376] -> w353
            tunnel: [w363 0.0 ("Angle Time Step (ms)")] -> w352
            event Timeout; "Start/pause": Value Change {
              n179 = event-data() -> ()  [unwired: 1 in, 2 out]
              n180 = call "Simulation Angle Step (SubVI).vi"("n"="Polynomial Degree", "N (Rot)"="Number of Rotations", "Final Angle"="Final Angle (deg)", "VISA Refnum in"=w365) -> ("Next Angle"=w367:dbl, "VISA Refnum out"=w366:refnum<visa-resource-name>, "Angle Time Step (ms)"=w363:dbl, "Rotation Complete?"=w360:bool)  [unwired: 3 in, 1 out]
              n181 = case shown="True" "Start/pause" {
                tunnel: [w373 100] -> w371
                tunnel: w370 -> [w373 _]
                frame False {
                }
                frame True {
                }
              }
              n182 = call "Move Absolute (SubVI).vi"("Move to Angle"=w367, "VISA Refnum in"=w366) -> ("New Angle"=→"Current Angle":dbl, "VISA Refnum out"=w364:refnum<visa-resource-name>)  [unwired: 7 in, 1 out]
            }
            event "Finish Rotation": Value Change {
              n183 = event-data() -> ()  [unwired: 1 in, 5 out]
            }
          }
          n184 = Wait (ms)(milliseconds to wait=w352) -> ()  [unwired: 1 out]
        }
        n185 = while {
          tunnel: w315 -> [w333]
          tunnel: w316 -> [w334]
          tunnel: [w334] -> _
          tunnel: [w333] -> w307
          shift-right: [w330] -> _
          shift-left: w309 -> [w331]
          tunnel: [w329] -> w311
          tunnel: w309 -> [w328]
          stop <- w329 stop-if-true
          # "SIMULATED STAGE MOVEMENT"
          n186 = event shown="[0] Timeout;  \"Start/Pause Stage\": Value Change" {
            selector: _ -> [_ _]
            dyn-events: _ -> [_ _]
            timeout: w331 -> [_ _]
            tunnel: [w344 "Finish Stage"] -> w329
            tunnel: [w346 w350] -> w330
            tunnel: w331 -> [_ w350]
            tunnel: [w345 0.0 ("Time Between Steps (ms)")] -> w332
            tunnel: w328 -> [w338 _]
            event Timeout; "Start/Pause Stage": Value Change {
              n187 = event-data() -> ()  [unwired: 1 in, 2 out]
              n188 = global write "Stage Global.vi" "Speed"("Speed (um/s)") -> ()
              n189 = global read "Stage Global.vi" "Position"() -> (w340:dbl)
              n190 = call "Slider Simulation Details (SubVI).vi"("Number of Steps"="Number of Steps") -> ("Time Between Steps (ms)"=w345:dbl, "Step Size (mm)"=w336:dbl)  [unwired: 9 in]
              n191 = global write "Stage Global.vi" "Final Position"("Final Position (mm)") -> ()
              n192 = Add(x=w340, y=w336) -> (x+y=w335:dbl)
              "Current Position (mm)" <- w335
              n193 = global read "Stage Global.vi" "Final Position"() -> (w337:dbl)
              n194 = case shown="True" "Start/Pause Stage" {
                tunnel: [w347 100] -> w346
                tunnel: w338 -> [w347 _]
                frame False {
                }
                frame True {
                }
              }
              n195 = global write "Stage Global.vi" "Position"(w335) -> ()
              n196 = Less Or Equal?(x=w337, y=w335) -> (x <= y?=w344:bool)
            }
            event "Finish Stage": Value Change {
              n197 = event-data() -> ()  [unwired: 1 in, 1 out]
            }
          }
          n198 = Wait (ms)(milliseconds to wait=w332) -> ()  [unwired: 1 out]
        }
        n199 = And(x=w312, y=w311) -> (x .and. y?=w313:bool)
        n200 = Not(x=w313) -> (.not. x?=w305:bool)
        n201 = local write "Finish Rotation"(w305) -> ()
        n202 = local write "Finish Stage"(w305) -> ()
        n203 = local write "Simulate?"(w305) -> ()
        n204 = Select(t=w306, s=TRUE, f=w307) -> (s? t:f=w298:errorcluster)
        n205 = property on="Scan Angles" class="Bool (strict)"(error in=w298, "DisabledEnum"=w300) -> (error out=w299:errorcluster)  [unwired: 1 in, 1 out]
        n206 = property on="Simulation" class="Bool (strict)"(error in=w299, "DisabledEnum"=w300) -> (error out=w319:errorcluster)  [unwired: 1 in, 1 out]
        n207 = property on="Scan" class="Bool (strict)"(error in=w319, "DisabledEnum"=w300) -> (error out=w322:errorcluster)  [unwired: 1 in, 1 out]
        n208 = property on="Go Home" class="Bool (strict)"(error in=w322, "DisabledEnum"=w300) -> (error out=w321:errorcluster)  [unwired: 1 in, 1 out]
        n209 = property on="Command" class="Bool (strict)"(error in=w321, "DisabledEnum"=w300) -> (error out=w320:errorcluster)  [unwired: 1 in, 1 out]
        n210 = local read "stop"() -> (w327:bool)
        "Simulate?" <- "Simulation"
      }
      event "stop": Value Change {
        n211 = event-data() -> ()  [unwired: 1 in, 5 out]
        n212 = local read "stop"() -> (w381:bool)
      }
    }
    n213 = local write "stop"("stop") -> ()
    n214 = Or(x="stop", y=w21) -> (x .or. y?=w24:bool)
  }
  n215 = call <instrlib>:"Close.vi"("error in (no error)"=w17, "VISA resource name"=w19) -> ("error out"=w16:errorcluster)  [unwired: 8 in, 1 out]
  n216 = call <vilib>:"General Error Handler.vi"("error in (no error)"=w16) -> ()  [unwired: 10 in, 5 out]
  "Calibrate?" <- w10
